vi "Configure Queue Connection.vi"(6 "timeout (500 ms)":i32=500, 8 "error in (no error)":errorcluster, 11 "Queue Name":string) -> (0 "error out":errorcluster, 3 "Connection.LocalQueue":refnum<class "Connection.LocalQueue.lvclass">)   [LabVIEW 2013, in "Connection.Queue_GOSPL.lvlib" / "Connection.LocalQueue.lvclass"]
uses:
  Connection.LocalQueue.lvclass
  Connection/Connection.lvclass/Connection.ctl
  Connection.LocalQueue.lvclass/Connection.LocalQueue.ctl
  Connection/Connection.lvclass
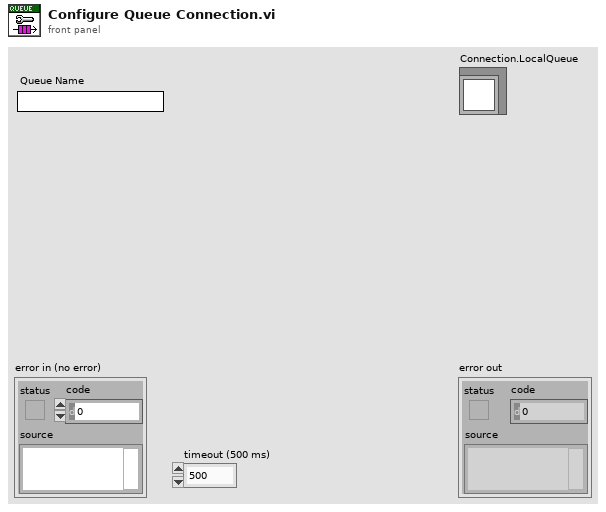
[diagram p1: front panel]
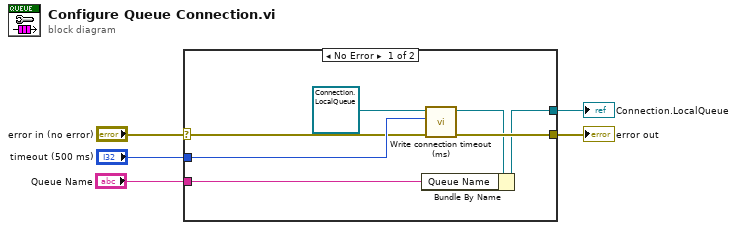
[diagram p0: block diagram]
diagram:
  n1 = case shown="No Error" "error in (no error)" {
    selector: "error in (no error)" -> [w11 w13]
    tunnel: [w10 w13] -> w4
    tunnel: [w8 _] -> w2
    tunnel: "timeout (500 ms)" -> [w12 _]
    tunnel: "Queue Name" -> [w7 _]
    frame No Error {
      n2 = call "Write connection timeout (ms).vi"("error in (no error)"=w11, "connection timeout (ms)"=w12, "Connection in"=refnum<class "Connection.LocalQueue.lvclass"> refnum ("Connection.LocalQueue")) -> ("error out"=w10:errorcluster, "Connection out"=w9:refnum<class "Connection.LocalQueue.lvclass">)  [unwired: 7 in]
      n3 = Bundle By Name(cluster=w9, "Queue Name"=w7) -> (w8:refnum<class "Connection.LocalQueue.lvclass">)
    }
    frame Error {
    }
  }
  "error out" <- w4
  "Connection.LocalQueue" <- w2
